vi "todos los modulos.vi"() -> ()   [LabVIEW 2010]
uses:
  <vilib>/sound2/lvsound2.llb/Sound Data Format.ctl
  <vilib>/addons/PixeLINK/Low Level Functions/CAMERA_FEATURES.llb/TDPU-CameraFeatures-PixelFormat.ctl
  <vilib>/sound2/lvsound2.llb/Sound Output Task ID.ctl
  <vilib>/vision/Image Controls.llb/IMAQ Image.ctl
panel:
  out "x-y":u8
  out "Contraste":u32
  out "Camara Funciona?":bool
  in  "Camera Parameters":T2 {"Pixel Format" items=["PIXEL_FORMAT_MONO8", "PIXEL_FORMAT_MONO16", "PIXEL_FORMAT_YUV422", "PIXEL_FORMAT_BAYER8_GRBG", "PIXEL_FORMAT_BAYER16_GRBG", "PIXEL_FORMAT_RGB24", "PIXEL_FORMAT_RGB48", "PIXEL_FORMAT_BAYER8_RGGB", "PIXEL_FORMAT_BAYER8_GBRG ", "PIXEL_FORMAT_BAYER8_BGGR ", "PIXEL_FORMAT_BAYER16_RGGB ", "PIXEL_FORMAT_BAYER16_GBRG", "PIXEL_FORMAT_BAYER16_BGGR", "PIXEL_FORMAT_RGB32"]}
  in  "Selector":u16(ring) items=["776002034"]
  in  "Streeam?":bool
  out "Image":T3(plugin-control)
  in  "Sound Controls":T5={"device ID"=0, "sound format"={"sample rate (S/s)"=44000.0, "number of channels"=2, "bits per sample"=16}, "time (ms)"=200.0}
  in  "Frecuencia":dbl
  out "Waveform Sound":waveform(dbl)(graph)
  in  "Sound?":bool
  in  "DAQ Controls":T6={"Minimum Value"=-10.0, "Maximum Value"=10.0, "Physical Channel"="Dev1/ao0", "DAQ Fs (S/s)"=10000.0} {"Minimum Value" min=-10.0 max=0.0; "Maximum Value" min=0.0 max=10.0}
  in  "Calibracion DAQ":T7
  out "Waveform DAQ":waveform(dbl)(graph)
  in  "tiempo (ms)":dbl
  in  "DAQ?":bool
  in  "stop":bool
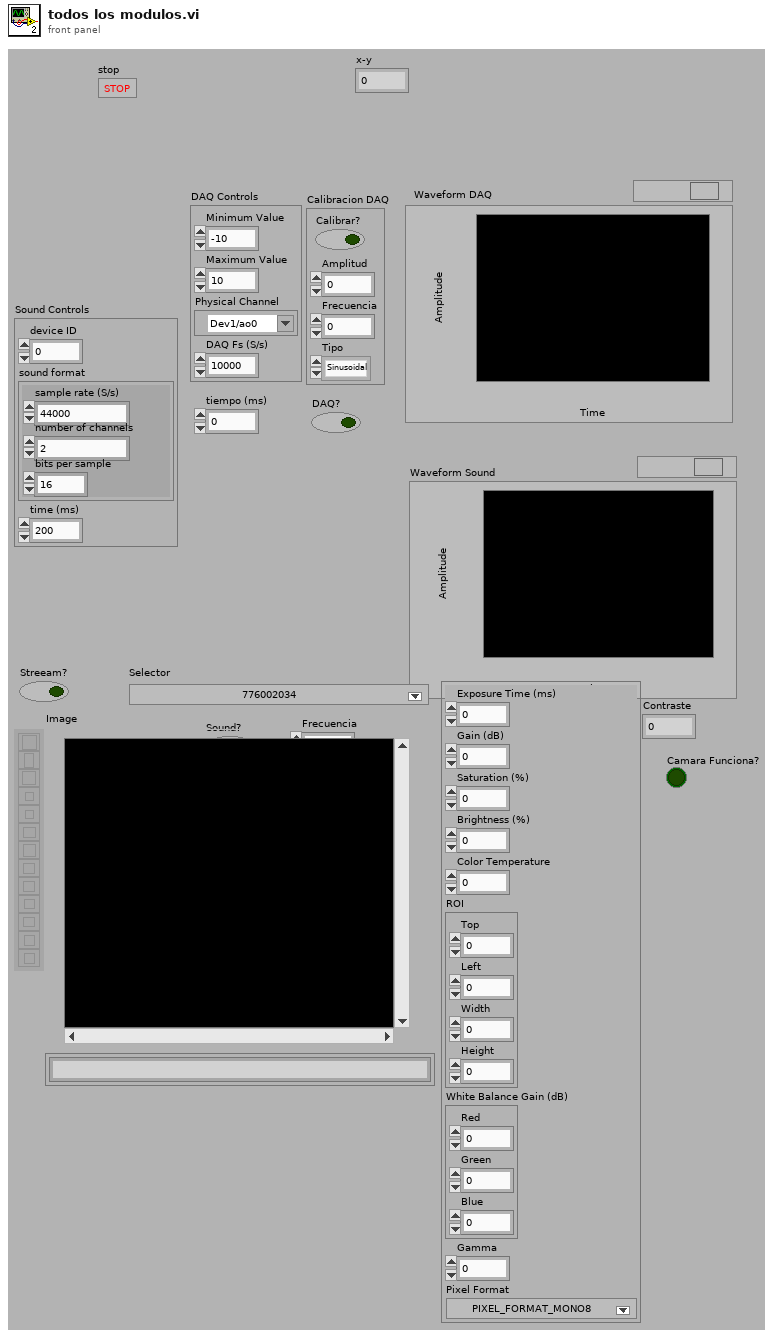
[diagram p1: front panel]
types:
  T1 = typedef "TDPU-CameraFeatures-PixelFormat.ctl" = u16
  T2 = cluster{"Exposure Time (ms)":u32, "Gain (dB)":dbl, "Saturation (%)":dbl, "Brightness (%)":dbl, "Color Temperature":dbl, "ROI":cluster{"Top":i32, "Left":i32, "Width":i32, "Height":i32}, "White Balance Gain (dB)":cluster{"Red":dbl, "Green":dbl, "Blue":dbl}, "Gamma":dbl, "Pixel Format":T1}
  T3 = typedef "IMAQ Image.ctl" = refnum<image>
  T4 = typedef "Sound Data Format.ctl" = cluster{"sample rate (S/s)":dbl, "number of channels":i32, "bits per sample":i32}
  T5 = cluster{"device ID":u32, "sound format":T4, "time (ms)":dbl}
  T6 = cluster{"Minimum Value":dbl, "Maximum Value":dbl, "Physical Channel":tag, "DAQ Fs (S/s)":dbl}
  T7 = cluster{"Calibrar?":bool, "Amplitud":dbl, "Frecuencia":dbl, "Tipo":enum16{"Sinusoidal", "Triangular", "Cuadrada"}}
  T8 = cluster{"hCamera":u32, "Error":errorcluster, "uSerialNumber OUT":u32}
  T9 = typedef "Sound Output Task ID.ctl" = u32
  T10 = cluster{"task ID":T9, "error":errorcluster, "sound format":T4}
  T11 = cluster{"DAQ Fs (S/s)":dbl, "task":refnum<k21>, "error":errorcluster, "Min Value":dbl, "Max Value":dbl}
  T12 = cluster{"DAQ Limits":cluster{"max":dbl, "min":dbl}, "Control Limits":cluster{"max":dbl, "min":dbl}}
  T13 = cluster{"hCamera":u32, "Error":errorcluster, "uSerialNumber":u32}
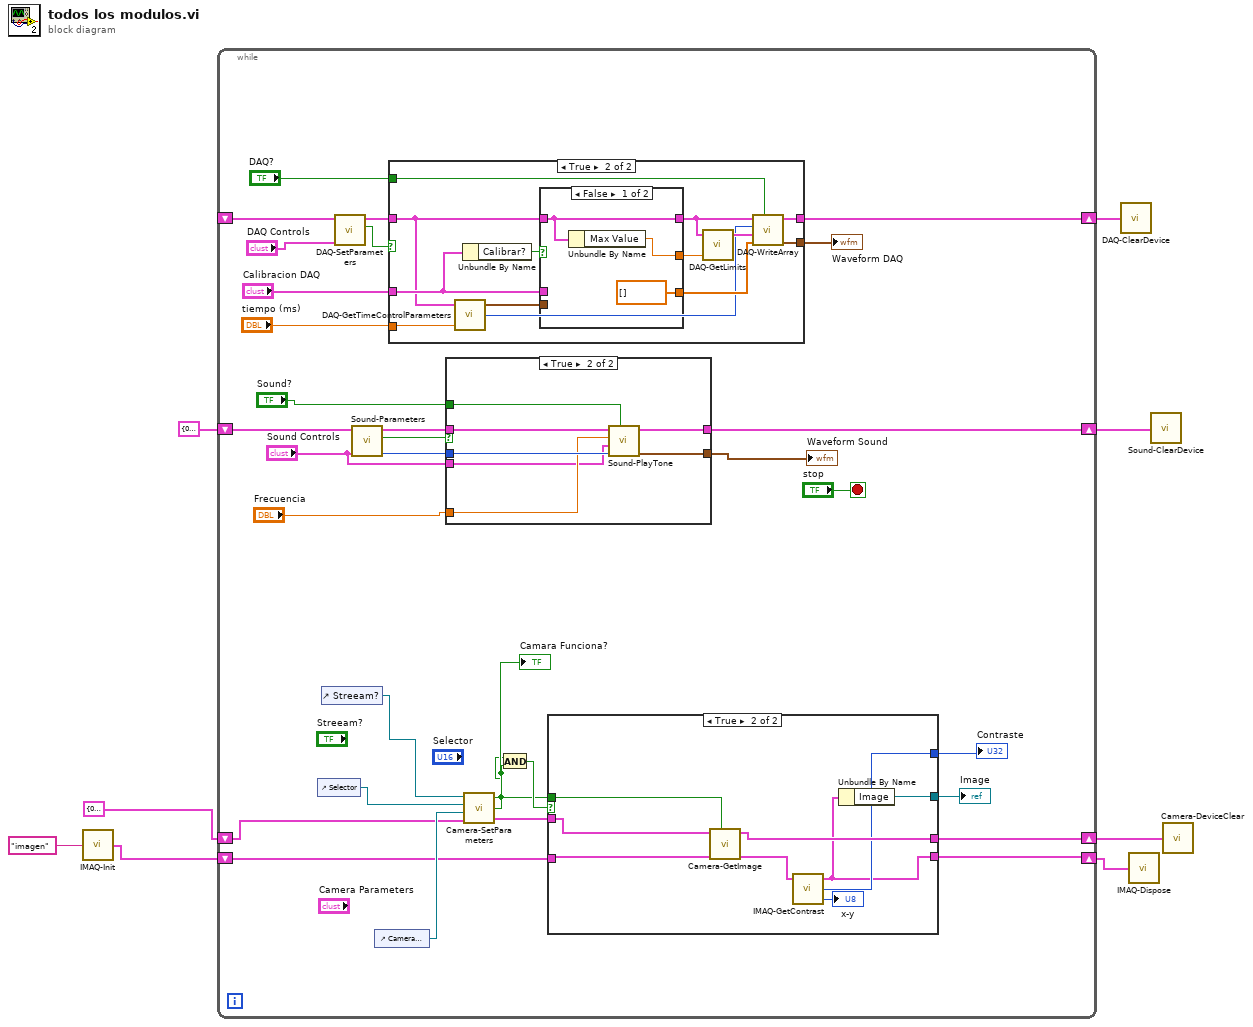
[diagram p0: block diagram]
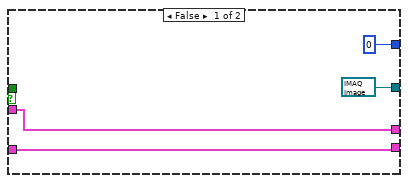
[diagram p2: hidden frame]
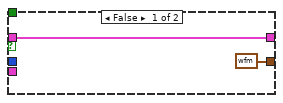
[diagram p3: hidden frame]
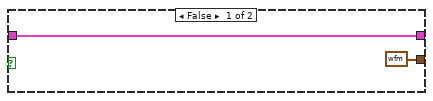
[diagram p4: hidden frame]
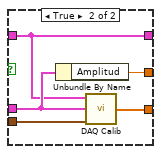
[diagram p5: hidden frame]
diagram:
  n1 = call "IMAQ-Init.vi"("Image Name"="imagen") -> ("Image Device IN"=w4:cluster{"Image":T3, "errorImage":errorcluster})
  n2 = while {
    shift-right: [w32] -> w6
    shift-left: _ -> [w33]
    shift-right: [w28] -> w7
    shift-left: T10 {"task ID"=0, "error"={"status"=TRUE, "code"=0, "source"=""}, "sound format"={"sample rate (S/s)"=0.0, "number of channels"=0, "bits per sample"=0}} ("Sound Device OUT") -> [w27]
    shift-right: [w13] -> w1
    shift-left: w4 -> [w17]
    shift-right: [w16] -> w2
    shift-left: T8 {"hCamera"=0, "Error"={"status"=FALSE, "code"=0, "source"=""}, "uSerialNumber OUT"=0} ("Camera Device  IN") -> [w15]
    stop <- "stop" stop-if-true
    n3 = control-ref of="Selector"() -> (w21:refnum<vi>)
    n4 = control-ref of="Streeam?"() -> (w19:refnum<vi>)
    n5 = call "DAQ-SetParameters.vi"("DAQ Controls"="DAQ Controls", "DAQ Device IN"=w33) -> ("En Funcionamiento?"=w26:bool, "DAQ Device OUT"=w38:T11)  [unwired: 4 in]
    n6 = call "Sound-Parameters.vi"("Sound Controls"="Sound Controls", "Sound Device IN"=w27) -> ("#samples"=w29:u32, "En funcionamiento?"=w25:bool, "Sound Device OUT"=w30:T10)  [unwired: 3 in]
    n7 = control-ref of="Camera Parameters"() -> (w20:refnum<vi>)
    n8 = case shown="True" w26 {
      tunnel: "DAQ?" -> [_ w75]
      tunnel: w38 -> [w64 w66]
      tunnel: [waveform(dbl) {"t0"=timestamp(0 s since 1904-01-01), "dt"=1.0, "Y"=[]} ("Waveform Graph") w72] -> w37
      tunnel: "Calibracion DAQ" -> [_ w68]
      tunnel: "tiempo (ms)" -> [_ w70]
      tunnel: [w64 w69] -> w32
      frame False {
      }
      frame True {
        n9 = call "DAQ-GetTimeControlParameters.vi"("tiempo (ms)"=w70, "DAQ Device IN"=w66) -> ("#samples"=w73:u32, "Time Control Parameters"=w74:cluster{"# samples":u32, "tiempos (ms)":dbl})  [unwired: 2 in]
        n10 = Unbundle By Name(w68) -> ("Calibrar?"=w67:bool)
        n11 = case shown="False" w67 {
          tunnel: [dbl[] [] ("Calibration OUT") w85] -> w77
          tunnel: w74 -> [_ w84]
          tunnel: w66 -> [w78 w81]
          tunnel: w68 -> [_ w83]
          tunnel: [w79 w82] -> w71
          tunnel: [w78 w81] -> w65
          frame False {
            n12 = Unbundle By Name(w78) -> ("Max Value"=w79:dbl)
          }
          frame True {
            n13 = Unbundle By Name(w83) -> ("Amplitud"=w82:dbl)
            n14 = call "DAQ Calib.vi"("Time Control Parameters"=w84, "Calibracion DAQ"=w83, "DAQ Device IN"=w81) -> ("Calibration OUT"=w85:dbl[])  [unwired: 1 in]
          }
        }
        n15 = call "DAQ-GetLimits.vi"("Amplitud"=w71, "DAQ Device IN"=w65) -> ("Limites"=w76:T12)  [unwired: 3 in]
        n16 = call "DAQ-WriteArray.vi"("DAQ?"=w75, "Control Array"=w77, "Limites"=w76, "#samples"=w73, "DAQ Device IN"=w65) -> ("Waveform Graph"=w72:waveform(dbl), "DAQ Device OUT"=w69:T11)  [unwired: 2 in]
      }
    }
    "Waveform DAQ" <- w37
    n17 = case shown="True" w25 {
      tunnel: [waveform(dbl) {"t0"=timestamp(0 s since 1904-01-01), "dt"=1.0, "Y"=[]} ("Waveform") w62] -> w31
      tunnel: w30 -> [w55 w61]
      tunnel: w29 -> [_ w60]
      tunnel: [w55 w59] -> w28
      tunnel: "Sound?" -> [_ w58]
      tunnel: "Frecuencia" -> [_ w57]
      tunnel: "Sound Controls" -> [_ w56]
      frame False {
      }
      frame True {
        n18 = call "Sound-PlayTone.vi"("sound?"=w58, "# samples"=w60, "Sound Controls"=w56, "Frecuencia"=w57, "Sound Device IN"=w61) -> ("Waveform"=w62:waveform(dbl), "Sound Device OUT"=w59:T10)  [unwired: 3 in]
      }
    }
    "Waveform Sound" <- w31
    n19 = call "Camera-SetParameters.vi"("Camera Device  IN"=w15, "Camera Parameters"=w20, "Selector"=w21, "Stream?"=w19) -> ("Camera Device OUT"=w18:T13, "Funciona?"=w11:bool, "Stream? OUT"=w10:bool)
    "Camara Funciona?" <- w11
    n20 = And(x=w10, y=w11) -> (x .and. y?=w12:bool)
    n21 = case shown="True" w12 {
      tunnel: w18 -> [w44 w52]
      tunnel: w10 -> [_ w53]
      tunnel: w17 -> [w43 w51]
      tunnel: [w44 w50] -> w16
      tunnel: [T3 refnum ("Image") w49] -> w14
      tunnel: [w43 w46] -> w13
      tunnel: [u32 0 ("Numeric") w48] -> w9
      frame False {
      }
      frame True {
        n22 = call "Camera-GetImage.vi"("Streeam"=w53, "Image Device IN"=w51, "Camera Device IN"=w52) -> ("Image Device OUT"=w47:cluster{"Image":T3, "errorImage":errorcluster}, "Camera Device OUT"=w50:T13)  [unwired: 4 in]
        n23 = call "IMAQ-GetContrast.vi"("Image Device IN"=w47) -> ("x-y"=→"x-y":u8, "Contraste"=w48:u8, "Image Device OUT"=w46:cluster{"Image":T3, "errorImage":errorcluster})  [unwired: 2 in]
        n24 = Unbundle By Name(w46) -> ("Image"=w49:T3)
      }
    }
    "Image" <- w14
    "Contraste" <- w9
  }
  n25 = call "DAQ-ClearDevice.vi"("DAQ Device IN"=w6) -> ()
  n26 = call "IMAQ-Dispose.vi"("Image Device IN"=w1) -> ()
  n27 = call "Sound-ClearDevice.vi"("Sound Device OUT"=w7) -> ()
  n28 = call "Camera-DeviceClear.vi"("Camera Device OUT"=w2) -> ()
